vi "get_path.vi"(9 "Message Prompt":string, 10 "operation (default: open/create)":T1(ring)=enum."open or create", 11 "Path In":path) -> (3 "Path out":string)   [LabVIEW 2012, in "LightPipes.lvlib"]
uses:
  Lightpipes.lvlib
panel:
  out "error out":errorcluster
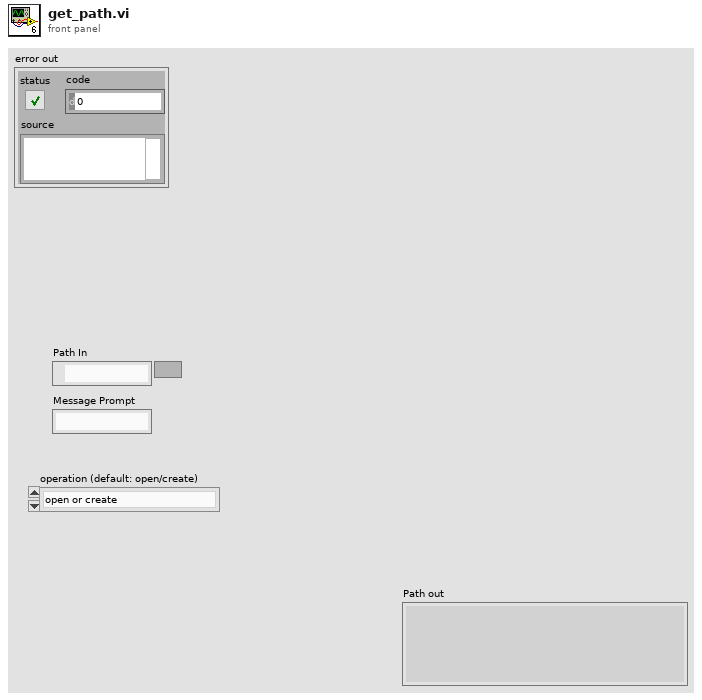
[diagram p1: front panel]
types:
  T1 = enum16{"open", "replace", "create", "open or create", "replace or create", "replace or create with confirmation"}
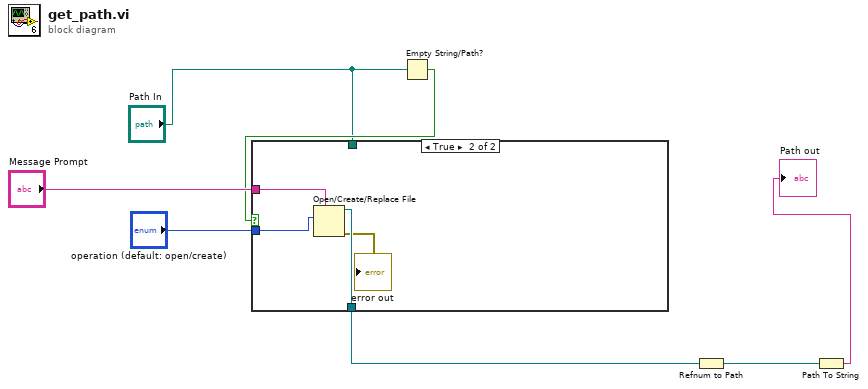
[diagram p0: block diagram]
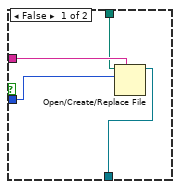
[diagram p2: hidden frame]
diagram:
  n1 = Empty String/Path?(string/path="Path In") -> (empty?=w5:bool)
  n2 = case shown="True" w5 {
    tunnel: "Message Prompt" -> [w11 w15]
    tunnel: "operation (default: open/create)" -> [w10 w14]
    tunnel: "Path In" -> [w9 _]
    tunnel: [w8 w13] -> w2
    frame False {
      n3 = Open/Create/Replace File(file path (use dialog)=w9, prompt=w11, operation (0:open)=w10) -> (refnum out=w8:refnum<file>)  [unwired: 3 in, 2 out]
    }
    frame True {
      n4 = Open/Create/Replace File(prompt=w15, operation (0:open)=w14) -> (refnum out=w13:refnum<file>, error out=→"error out":errorcluster)  [unwired: 4 in, 1 out]
    }
  }
  n5 = Refnum to Path(1:w2) -> (0:w3:path)
  n6 = Path To String(path=w3) -> (string=→"Path out":string)
